vi "discharging.vi"(0 "E":dbl, 1 "R":dbl, 2 "C":dbl) -> (6 "TIME = 3":dbl format="%#_3e", 7 "VC T = 4":dbl format="%#_3e", 8 "TIME = 2":dbl format="%#_3e", 9 "VC T = 3":dbl format="%#_3e", 10 "Time Const":dbl, 11 "VC T = 2":dbl format="%#_3e", 12 "TIME = 4":dbl format="%#_3e", 13 "VC T = 1":dbl format="%#_3e", 14 "TIME = 1":dbl format="%#_3e", 15 "TIME = 5":dbl format="%#_3e", 16 "TIME = 0":dbl format="%#_3e", 17 "VC T = 5":dbl format="%#_3e", 18 "VC T = 0":dbl format="%#_3e")   [LabVIEW 2018]
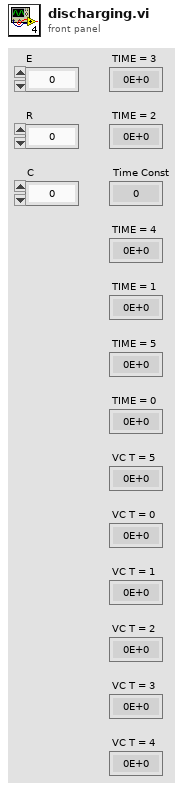
[diagram p1: front panel]
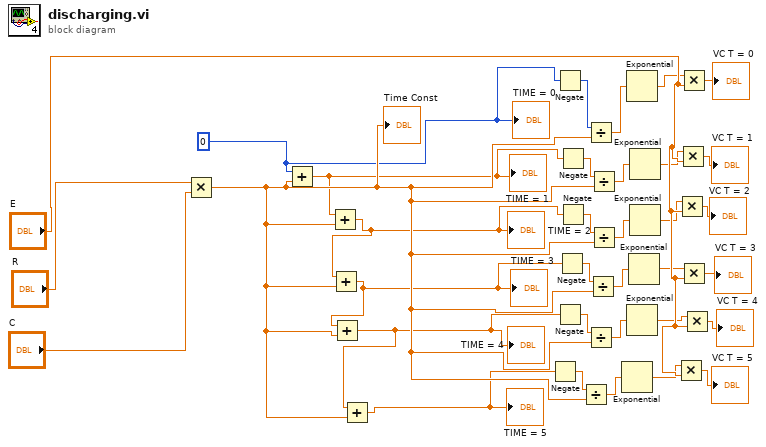
[diagram p0: block diagram]
diagram:
  w15 = 0
  n1 = Multiply(x="R", y="C") -> (x*y=w21:dbl)
  "Time Const" <- w21
  n2 = Add(x=w15, y=w21) -> (x+y=w16:dbl)
  "TIME = 1" <- w16
  n3 = Add(x=w16, y=w21) -> (x+y=w17:dbl)
  "TIME = 2" <- w17
  n4 = Add(x=w17, y=w21) -> (x+y=w18:dbl)
  "TIME = 3" <- w18
  n5 = Add(x=w18, y=w21) -> (x+y=w19:dbl)
  "TIME = 4" <- w19
  n6 = Add(x=w19, y=w21) -> (x+y=w20:dbl)
  "TIME = 5" <- w20
  n7 = Negate(x=w20) -> (-x=w13:dbl)
  n8 = Negate(x=w15) -> (-x=w3:i32)
  n9 = Negate(x=w19) -> (-x=w11:dbl)
  n10 = Negate(x=w18) -> (-x=w9:dbl)
  n11 = Negate(x=w16) -> (-x=w5:dbl)
  n12 = Negate(x=w17) -> (-x=w7:dbl)
  n13 = Divide(x=w13, y=w21) -> (x/y=w14:dbl)
  n14 = Divide(x=w3, y=w21) -> (x/y=w4:dbl)
  n15 = Divide(x=w11, y=w21) -> (x/y=w12:dbl)
  n16 = Divide(x=w9, y=w21) -> (x/y=w10:dbl)
  n17 = Divide(x=w5, y=w21) -> (x/y=w6:dbl)
  n18 = Divide(x=w7, y=w21) -> (x/y=w8:dbl)
  n19 = Exponential(1:w14) -> (0:w23:dbl)
  n20 = Exponential(1:w4) -> (0:w22:dbl)
  n21 = Exponential(1:w12) -> (0:w24:dbl)
  n22 = Exponential(1:w10) -> (0:w25:dbl)
  n23 = Exponential(1:w6) -> (0:w27:dbl)
  n24 = Exponential(1:w8) -> (0:w26:dbl)
  n25 = Multiply(x=w23, y="E") -> (x*y=→"VC T = 5":dbl)
  n26 = Multiply(x=w26, y="E") -> (x*y=→"VC T = 2":dbl)
  n27 = Multiply(x=w27, y="E") -> (x*y=→"VC T = 1":dbl)
  n28 = Multiply(x=w22, y="E") -> (x*y=→"VC T = 0":dbl)
  n29 = Multiply(x=w25, y="E") -> (x*y=→"VC T = 3":dbl)
  n30 = Multiply(x=w24, y="E") -> (x*y=→"VC T = 4":dbl)
  "TIME = 0" <- w15
